vi "Write Path.vi"(8 "error in (no error)":errorcluster, 10 "Path":path, 11 "Grid in":refnum<class "Grid.lvclass">) -> (0 "error out":errorcluster, 3 "Grid out":refnum<class "Grid.lvclass">)   [LabVIEW 2013, in "Grid.lvclass"]
uses:
  Grid.lvclass
  Grid.lvclass/Grid.ctl
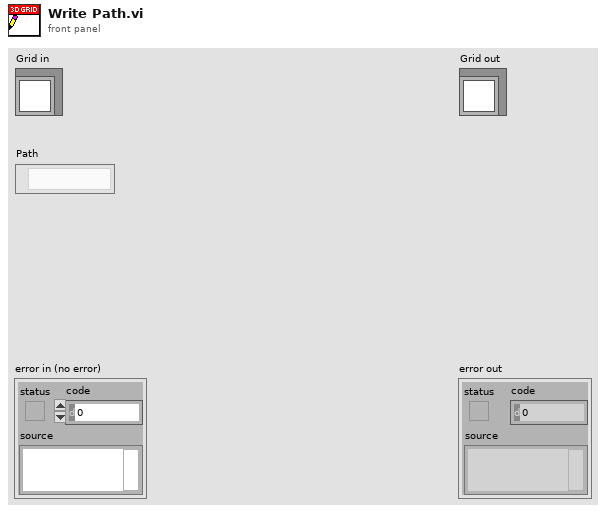
[diagram p1: front panel]
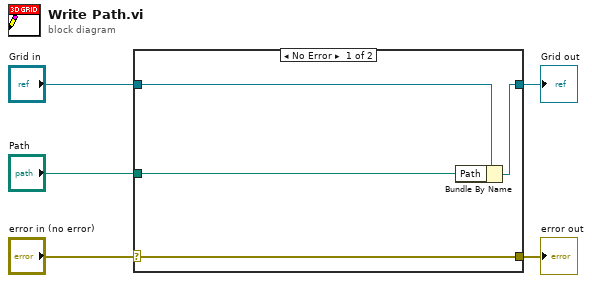
[diagram p0: block diagram]
diagram:
  n1 = case shown="No Error" "error in (no error)" {
    selector: "error in (no error)" -> [w9 w10]
    tunnel: [w9 w10] -> w4
    tunnel: [w7 w11] -> w2
    tunnel: "Grid in" -> [w8 w11]
    tunnel: "Path" -> [w6 _]
    frame No Error {
      n2 = Bundle By Name(cluster=w8, "Path"=w6) -> (w7:refnum<class "Grid.lvclass">)
    }
    frame Error {
    }
  }
  "error out" <- w4
  "Grid out" <- w2
